vi "addPubSub.vi"(9 "PubSub":T1, 11 "ROS_Master in":refnum<class "ROS_Master.lvclass">) -> (3 "ROS_Master out":refnum<class "ROS_Master.lvclass">)   [LabVIEW 2012, in "ROS_Master.lvclass"]
uses:
  <userlib>/ROSforLV/ROS/Code/ROS_Master/ROS_Master.lvclass
  <userlib>/ROSforLV/ROS/Code/ROS_Master/ROS_Master.lvclass/ROS_Master.ctl
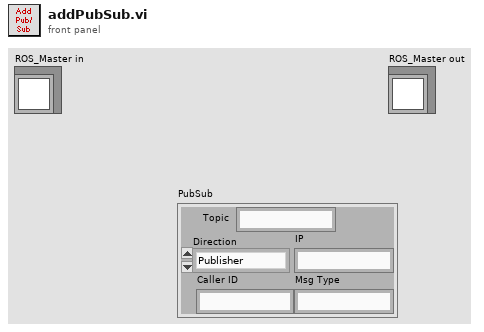
[diagram p1: front panel]
types:
  T1 = cluster{"Caller ID":string, "IP":string, "Msg Type":string, "Direction":enum16{"Publisher", "Subscriber"}, "Topic":string}
  T2 = cluster{"Name":string, "PubSubs":cluster{"Caller ID":string, "IP":string, "Msg Type":string, "Direction":enum16{"Publisher", "Subscriber"}, "Topic":string}[]}[]
  T3 = cluster{"Caller ID":string, "IP":string, "Msg Type":string, "Direction":enum16{"Publisher", "Subscriber"}, "Topic":string}[]
  T4 = cluster{"Topic":string, cluster{"Caller ID":string, "IP":string, "Msg Type":string, "Direction":enum16{"Publisher", "Subscriber"}, "Topic":string}[]}
  T5 = cluster{"Name":string, "PubSubs":cluster{"Caller ID":string, "IP":string, "Msg Type":string, "Direction":enum16{"Publisher", "Subscriber"}, "Topic":string}[]}
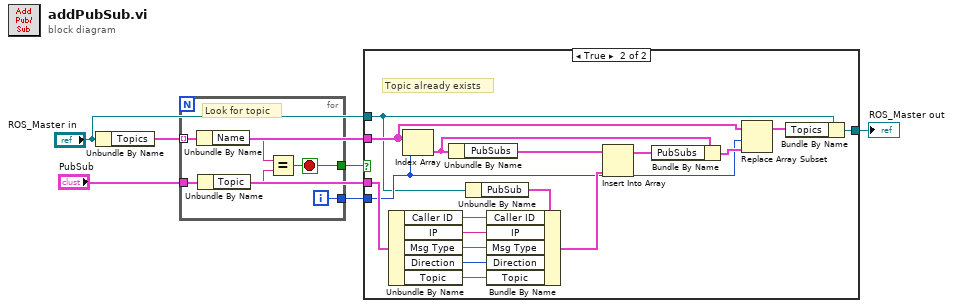
[diagram p0: block diagram]
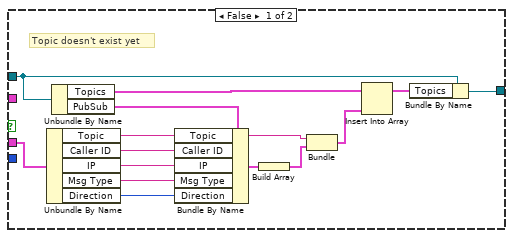
[diagram p2: hidden frame]
diagram:
  n1 = Unbundle By Name("ROS_Master in") -> ("Topics"=w4:T2)
  n2 = for {
    tunnel: w4 -> [w12] mode=indexing
    tunnel: "PubSub" -> [w11]
    tunnel: [w8] -> w6
    tunnel: [w7] -> w5
    i -> [w7]
    stop <- w8 stop-if-true
    # "Look for topic"
    n3 = Unbundle By Name(w12) -> ("Name"=w10:string)
    n4 = Unbundle By Name(w11) -> ("Topic"=w9:string)
    n5 = Equal?(x=w10, y=w9) -> (x = y?=w8:bool)
  }
  n6 = case shown="True" w6 {
    tunnel: "PubSub" -> [w22 w42]
    tunnel: w5 -> [_ w33]
    tunnel: w4 -> [_ w34]
    tunnel: "ROS_Master in" -> [w17 w31]
    tunnel: [w15 w29] -> w3
    frame False {
      # "Topic doesn't exist yet"
      n7 = Unbundle By Name(w22) -> ("Topic"=w13:string, "Caller ID"=w25:string, "IP"=w24:string, "Msg Type"=w23:string, "Direction"=w14:enum16{"Publisher", "Subscriber"})
      n8 = Unbundle By Name(w17) -> ("Topics"=w19:T2, "PubSub"=w26:T1)
      n9 = Bundle By Name(cluster=w26, "Topic"=w13, "Caller ID"=w25, "IP"=w24, "Msg Type"=w23, "Direction"=w14) -> (w21:T1)
      n10 = Build Array(w21) -> (w20:T3)
      n11 = Bundle("Topic"=w13, w20) -> (w18:T4)  [unwired: 1 in]
      n12 = Insert Into Array(array=w19, new element=w18) -> (w16:T2)  [unwired: 1 in]
      n13 = Bundle By Name(cluster=w17, "Topics"=w16) -> (w15:refnum<class "ROS_Master.lvclass">)
    }
    frame True {
      # "Topic already exists"
      n14 = Unbundle By Name(w42) -> ("Caller ID"=w41:string, "IP"=w40:string, "Msg Type"=w39:string, "Direction"=w28:enum16{"Publisher", "Subscriber"}, "Topic"=w27:string)
      n15 = Index Array(array=w34, index=w33) -> (element=w37:T5)
      n16 = Unbundle By Name(w37) -> ("PubSubs"=w43:T3)
      n17 = Unbundle By Name(w31) -> ("PubSub"=w32:T1)
      n18 = Bundle By Name(cluster=w32, "Caller ID"=w41, "IP"=w40, "Msg Type"=w39, "Direction"=w28, "Topic"=w27) -> (w38:T1)
      n19 = Insert Into Array(array=w43, new element=w38) -> (w36:T3)  [unwired: 1 in]
      n20 = Bundle By Name(cluster=w37, "PubSubs"=w36) -> (w35:T5)
      n21 = Replace Array Subset(array=w34, new element=w35, index=w33) -> (w30:T2)
      n22 = Bundle By Name(cluster=w31, "Topics"=w30) -> (w29:refnum<class "ROS_Master.lvclass">)
    }
  }
  "ROS_Master out" <- w3
